vi "Date_n_time.vi"() -> (1 "time string":string, 2 "Date+time (YYYYMMDD-HHMMSS)":string, 3 "date string":string)   [LabVIEW 2019]
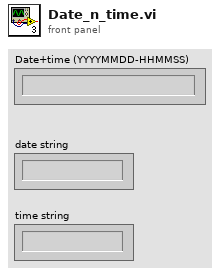
[diagram p1: front panel]
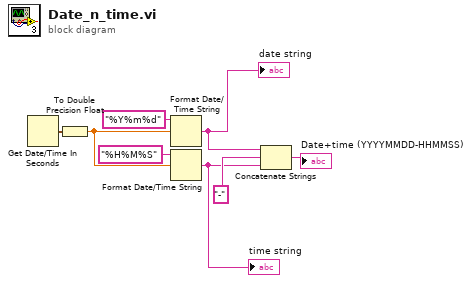
[diagram p0: block diagram]
diagram:
  n1 = Get Date/Time In Seconds() -> (seconds since 1Jan1904=w7:timestamp)
  n2 = To Double Precision Float(number=w7) -> (double precision float=w5:dbl)
  n3 = Format Date/Time String(time format string (%c)="%Y%m%d", seconds (now)=w5) -> (date/time string=w1:string)  [unwired: 1 in]
  "date string" <- w1
  n4 = Format Date/Time String(time format string (%c)="%H%M%S", seconds (now)=w5) -> (date/time string=w4:string)  [unwired: 1 in]
  "time string" <- w4
  n5 = Concatenate Strings(w1, "-" ("string"), w4) -> (→"Date+time (YYYYMMDD-HHMMSS)":string)
